vi "sv_Compute Low Pass Filter Denominator.vi"(0 "w":dbl, 7 "s":cdb, 11 "Q":dbl=0.7071067811865475 format="%#_26g") -> (4 "result":cdb)   [LabVIEW 2017]
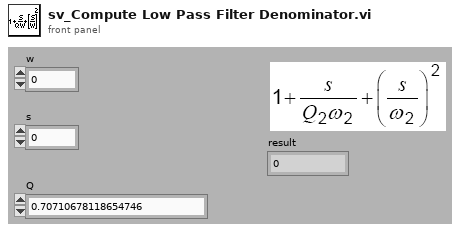
[diagram p1: front panel]
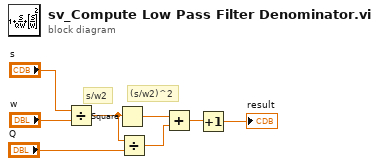
[diagram p0: block diagram]
diagram:
  # "(s/w2)^2"
  # "s/w2"
  n1 = Divide(x="s", y="w") -> (x/y=w6:cdb)
  n2 = Square(x=w6) -> (x^2=w7:cdb)
  n3 = Divide(x=w6, y="Q") -> (x/y=w8:cdb)
  n4 = Add(x=w7, y=w8) -> (x+y=w5:cdb)
  n5 = Increment(x=w5) -> (x+1=→"result":cdb)
